vi "Terminate.vi"(6 "Teller":refnum<class "Teller.lvclass">, 9 "Error":errorcluster, 10 "Actor":refnum<class "Actor.lvclass">, 11 "Terminate in":refnum<class "Terminate.lvclass">) -> (0 "Error out":errorcluster, 3 "Terminate out":refnum<class "Terminate.lvclass">)   [LabVIEW 2025, in "jettl.lvlib" / "Terminate Msg.lvlib" / "Terminate.lvclass"]
uses:
  Terminate.lvclass
  Actor/Actor/Actor.lvclass
  Teller/Teller/Teller.lvclass
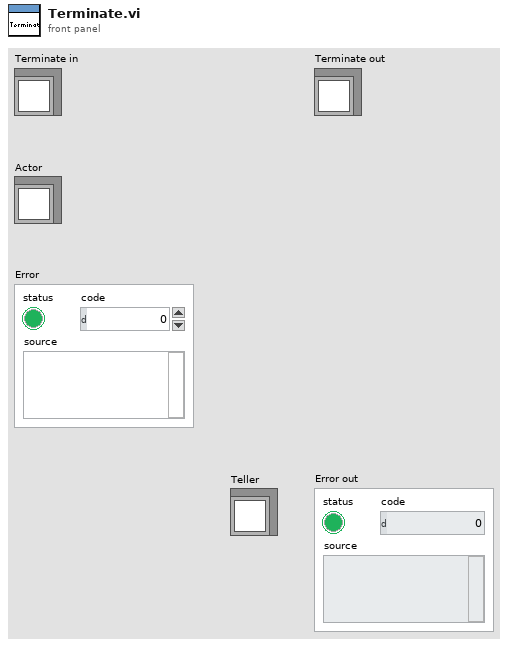
[diagram p1: front panel]
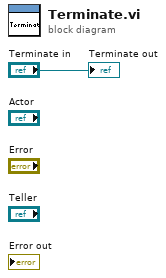
[diagram p0: block diagram]
diagram:
  "Terminate out" <- "Terminate in"
